vi "DevicesDashboard.vi"() -> ()   [LabVIEW 2019]
uses:
  RIOData--cluster.ctl
  PicoData.ctl
  df630f77-700f-42c8-8b14-ed8bcaa39713.vi
  a087fea8-a487-4c1c-8a8b-15f205e78756.vi
  bb14a938-b648-4f31-b7d9-8aca462ae9c1.vi
  <vilib>/JDP Science/JSONtext/JSON text to Variant.vi
  <vilib>/JDP Science/JSONtext/LVClass Serializer/JSONtext LVClass Serializer.lvclass
  <vilib>/PantherLAB/Firebase API/PantherLAB_lib_firebase.lvclass
  Shared.lvlib
panel:
  out "RIO Juan":T1
  out "Pico Enrique":T2
  in  "Password":string="123456"
  in  "Email":string="enrique.noe@gmail.com"
  in  "Log In":bool
  out "RIO Enrique":T1
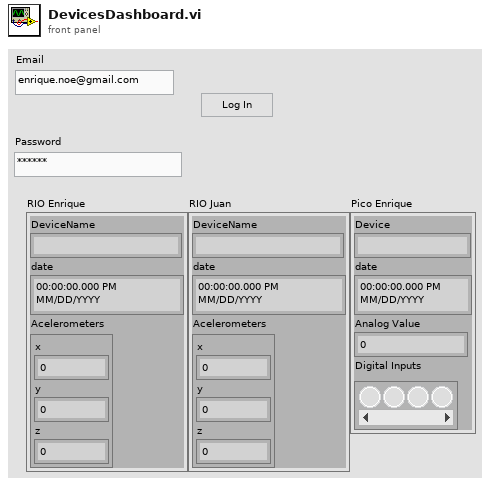
[diagram p1: front panel]
types:
  T1 = typedef "Shared.lvlib/RIOData--cluster.ctl" = cluster{"DeviceName":string, "date":timestamp, "Acelerometers":cluster{"x":dbl, "y":dbl, "z":dbl}}
  T2 = typedef "Shared.lvlib/PicoData.ctl" = cluster{"Device":string, "date":timestamp, "Analog Value":u16, "Digital Inputs":bool[]}
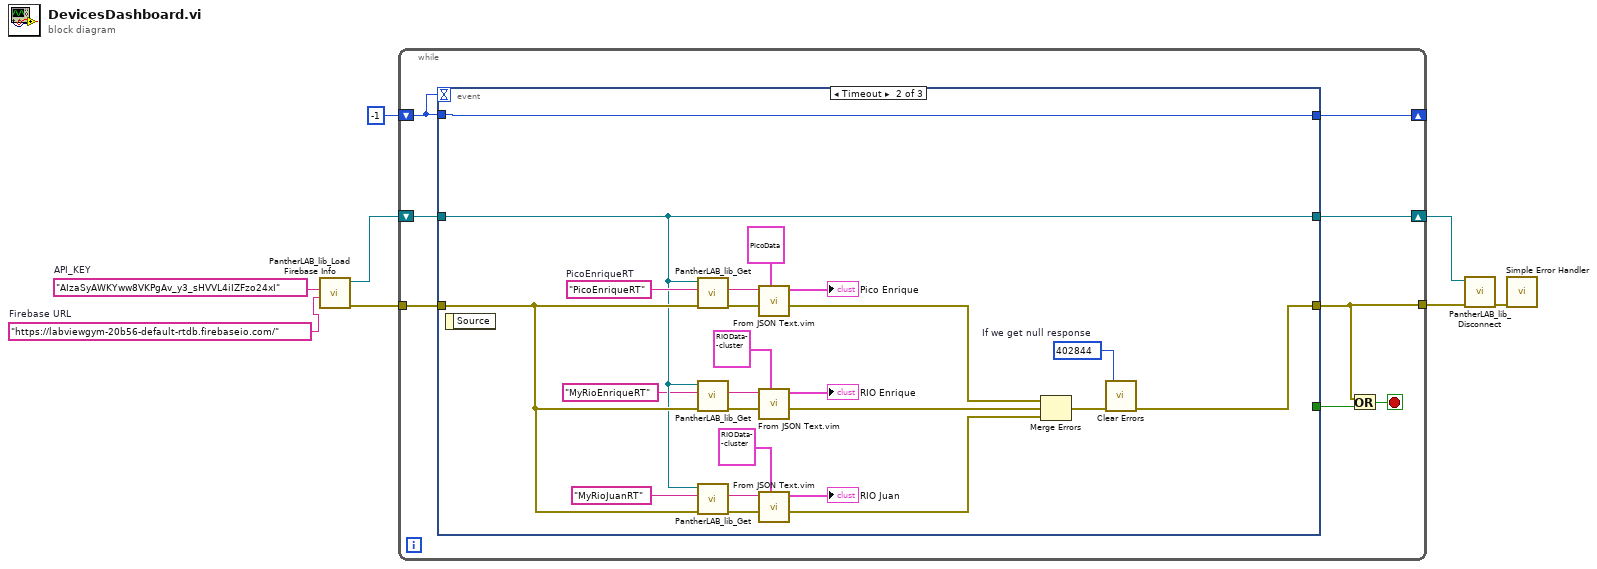
[diagram p0: block diagram]
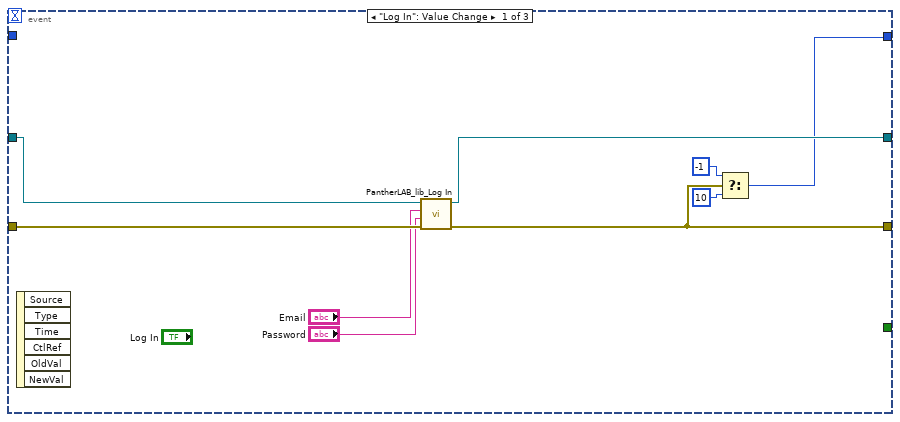
[diagram p2: hidden frame]
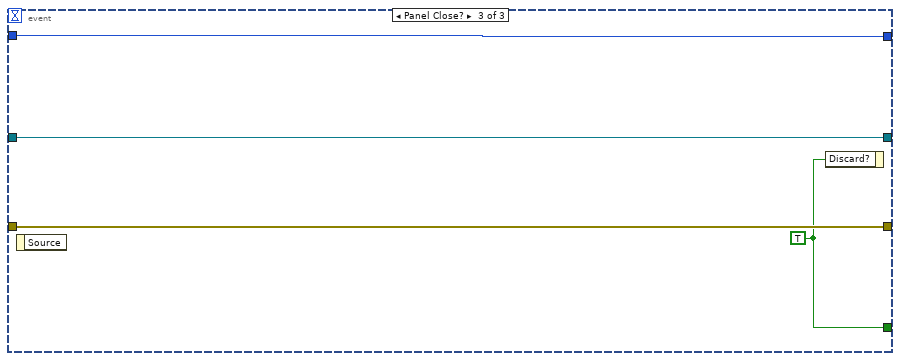
[diagram p3: hidden frame]
diagram:
  w3 = "AIzaSyAWKYww8VKPgAv_y3_sHVVL4iIZFzo24xI"  # API_KEY
  w2 = "https://labviewgym-20b56-default-rtdb.firebaseio.com/"  # Firebase URL
  n1 = call <vilib>:"PantherLAB_lib_Load Firebase Info.vi"("Firebase URL"=w2, "API_KEY"=w3) -> ("error out"=w6:errorcluster, "firebase out"=w4:refnum<class "PantherLAB_lib_firebase.lvclass">)  [unwired: 8 in]
  n2 = while {
    tunnel: w6 -> [w16]
    tunnel: [w15] -> w7
    shift-right: [w11] -> w5
    shift-left: w4 -> [w12]
    shift-right: [w10] -> _
    shift-left: -1 -> [w9]
    stop <- w13 stop-if-true
    n3 = event shown="[1] Timeout" {
      selector: _ -> [_ _ _]
      dyn-events: _ -> [_ _ _]
      timeout: w9 -> [_ _ _]
      tunnel: w16 -> [w25 w44 w53]
      tunnel: [w24 w45 w53] -> w15
      tunnel: [_ _ w51] -> w14
      tunnel: w12 -> [w20 w29 w52]
      tunnel: [w21 w29 w52] -> w11
      tunnel: [w17 w40 w50] -> w10
      tunnel: w9 -> [_ w40 w50]
      event "Log In": Value Change {
        n4 = event-data() -> ()  [unwired: 1 in, 6 out]
        n5 = call-dynamic "PantherLAB_lib_Log In.vi"("error in"=w25, "password"="Password", "email"="Email", "firebase in"=w20) -> ("error out"=w24:errorcluster, "firebase out"=w21:refnum<class "PantherLAB_lib_firebase.lvclass">)  [unwired: 6 in]
        n6 = Select(t=-1, s=w24, f=10) -> (s? t:f=w17:i32)
      }
      event Timeout {
        w26 = 402844  # If we get null response
        w30 = "PicoEnriqueRT"  # PicoEnriqueRT
        n7 = event-data() -> ()  [unwired: 1 in, 1 out]
        n8 = call-dynamic "PantherLAB_lib_Get.vi"("error in"=w44, "endPoint"=w30, "firebase in"=w29) -> ("error out"=w48:errorcluster, "Json String"=w38:string)  [unwired: 7 in]
        n9 = call-dynamic "PantherLAB_lib_Get.vi"("error in"=w44, "endPoint"="MyRioEnriqueRT", "firebase in"=w29) -> ("error out"=w49:errorcluster, "Json String"=w39:string)  [unwired: 7 in]
        n10 = call-dynamic "PantherLAB_lib_Get.vi"("error in"=w44, "endPoint"="MyRioJuanRT", "firebase in"=w29) -> ("error out"=w47:errorcluster, "Json String"=w33:string)  [unwired: 7 in]
        n11 = call "From JSON Text.vim"("Data Type and Default Value"=T2 {"Device"="", "date"=timestamp(0 s since 1904-01-01), "Analog Value"=0, "Digital Inputs"=[]} ("output cluster"), "error in (no error)"=w48, "JSON"=w38) -> ("error out"=w42:errorcluster, "Data out"=→"Pico Enrique":T2)  [unwired: 7 in]
        n12 = call "From JSON Text.vim"("Data Type and Default Value"=T1 {"DeviceName"="", "date"=timestamp(0 s since 1904-01-01), "Acelerometers"={"x"=0.0, "y"=0.0, "z"=0.0}} ("Array"), "error in (no error)"=w49, "JSON"=w39) -> ("error out"=w41:errorcluster, "Data out"=→"RIO Enrique":T1)  [unwired: 7 in]
        n13 = call "From JSON Text.vim"("Data Type and Default Value"=T1 {"DeviceName"="", "date"=timestamp(0 s since 1904-01-01), "Acelerometers"={"x"=0.0, "y"=0.0, "z"=0.0}} ("Array"), "error in (no error)"=w47, "JSON"=w33) -> ("error out"=w46:errorcluster, "Data out"=→"RIO Juan":T1)  [unwired: 7 in]
        n14 = Merge Errors(w42, w41, w46) -> (w43:errorcluster)
        n15 = call <vilib>:"Clear Errors.vi"("error in (no error)"=w43, "specific error code to clear (0: all)"=w26) -> ("error out"=w45:errorcluster)  [unwired: 4 in, 1 out]
      }
      event Panel Close? {
        w51 = TRUE ("Discard?")
        n16 = event-data() -> ()  [unwired: 1 in, 1 out]
        n17 = event-data("Discard?"=w51) -> ()  [unwired: 1 in, 1 out]
      }
    }
    n18 = Or(x=w15, y=w14) -> (x .or. y?=w13:bool)
  }
  n19 = call-dynamic "PantherLAB_lib_Disconnect.vi"("error in"=w7, "firebase in"=w5) -> ("error out"=w8:errorcluster)  [unwired: 9 in]
  n20 = call <vilib>:"Simple Error Handler.vi"("error in (no error)"=w8) -> ()  [unwired: 4 in, 5 out]
